vi "Check Waveform Property Name.vi"(7 "Property Name":string[](array[string]), 8 "error in (no error)":errorcluster, 9 "Group Name":string, 10 "Channel Name":string, 11 "TDMS File In":refnum<k34>) -> (0 "error out":errorcluster, 3 "TDMS File Out":refnum<k34>)   [LabVIEW 2013, in "Agilent 90000 Series.lvlib"]
doc: "Checks whether the TDMS file has specified property name. If not, it will return a specific error."
uses:
  Agilent 90000 Series.lvlib
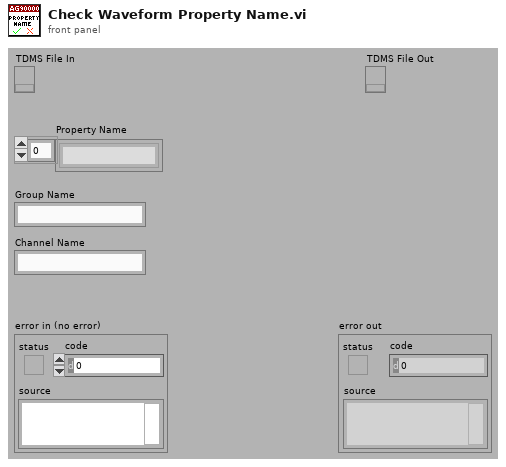
[diagram p1: front panel]
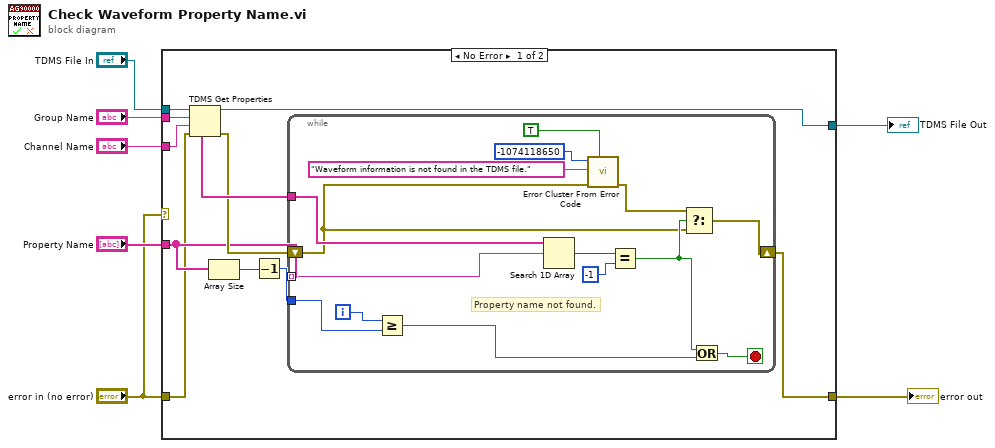
[diagram p0: block diagram]
diagram:
  n1 = case shown="No Error" "error in (no error)" {
    tunnel: "TDMS File In" -> [w18 w34]
    tunnel: "Group Name" -> [w17 _]
    tunnel: "Channel Name" -> [w16 _]
    tunnel: "Property Name" -> [w13 _]
    tunnel: [w10 w35] -> w3
    tunnel: "error in (no error)" -> [w9 w35]
    tunnel: [w8 w34] -> w2
    frame No Error {
      n2 = TDMS Get Properties(8:w9, 9:w16, 10:w17, 11:w18) -> (0:w14:errorcluster, 3:w8:refnum<k34>, 6:w15:string[])  [unwired: 2 in, 3 out]
      n3 = Array Size(array=w13) -> (size(s)=w12:i32)
      n4 = Decrement(x=w12) -> (x-1=w11:i32)
      n5 = while {
        tunnel: w15 -> [w31]
        tunnel: w13 -> [w30] mode=indexing
        tunnel: w11 -> [w32]
        shift-right: [w20] -> w10
        shift-left: w14 -> [w19]
        i -> [w33]
        stop <- w26 stop-if-true
        # "Property name not found."
        n6 = Greater Or Equal?(x=w33, y=w32) -> (x >= y?=w27:bool)
        n7 = Search 1D Array(1D array=w31, element=w30) -> (index of element=w29:i32)  [unwired: 1 in]
        n8 = call <vilib>:"Error Cluster From Error Code.vi"("show call chain? (False)"=TRUE, "error in (no error)"=w19, "error message (\"\")"="Waveform information is not found in the TDMS file." ("error message (\"\")"), "error code (0)"=-1074118650) -> ("error out"=w21:errorcluster)  [unwired: 5 in]
        n9 = Equal?(x=w29, y=-1) -> (x = y?=w22:bool)
        n10 = Select(t=w21, s=w22, f=w19) -> (s? t:f=w20:errorcluster)
        n11 = Or(x=w22, y=w27) -> (x .or. y?=w26:bool)
      }
    }
    frame Error {
    }
  }
  "error out" <- w3
  "TDMS File Out" <- w2
